vi "EXPIREAT.vi"(0 "refnum in":refnum<vi>, 1 "Key":string, 5 "Timestamp":string, 11 "error in":errorcluster) -> (4 "refnum out":refnum<vi>, 6 "Data":T1, 15 "error out":errorcluster)   [LabVIEW 2020]
uses:
  SubVIs/Controls/redis-data.ctl
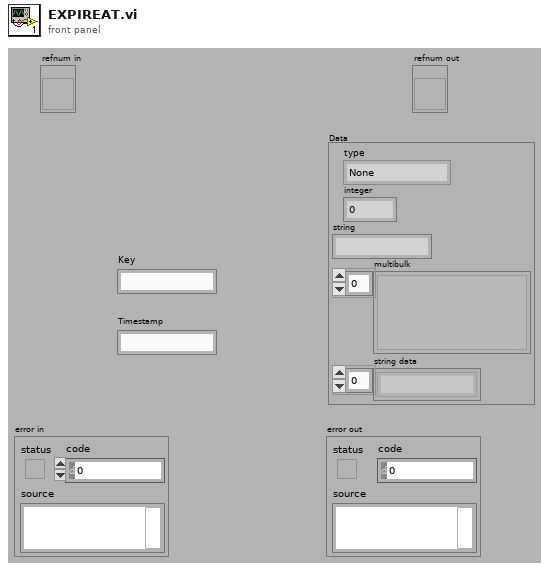
[diagram p1: front panel]
types:
  T1 = typedef "redis-data.ctl" = cluster{"type":enum16{"None", "Error", "Status", "Nil", "Integer", "String", "Multibulk"}, "integer":i64, "string":string, "multibulk":variant[], "string data":string[]}
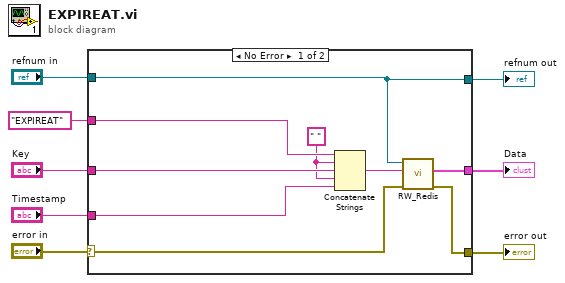
[diagram p0: block diagram]
diagram:
  n1 = case shown="No Error" "error in" {
    selector: "error in" -> [w15 w19]
    tunnel: "Key" -> [w12 _]
    tunnel: "EXPIREAT" -> [w17 _]
    tunnel: "refnum in" -> [w9 w18]
    tunnel: [w14 w19] -> w6
    tunnel: [w13 _] -> w2
    tunnel: "Timestamp" -> [w10 _]
    tunnel: [w9 w18] -> w3
    frame No Error {
      w11 = " "
      n2 = Concatenate Strings(w17, w11, w12, w11, w10) -> (w16:string)
      n3 = call "RW_Redis.vi"("error in"=w15, "command"=w16, "refnum"=w9) -> ("error out"=w14:errorcluster, "Data"=w13:T1)  [unwired: 7 in]
    }
    frame Error {
    }
  }
  "error out" <- w6
  "refnum out" <- w3
  "Data" <- w2
